vi "BUFMGR_API.vi"(0 "modpath":path, 7 "Cmd":string, 11 "error in":errorcluster) -> (4 "ImmedReplyString":string, 15 "error out":errorcluster)   [LabVIEW 2016]
uses:
  DBSHAND/private/vis/DatabaseHand_Element_Set(bool).vi
panel:
  out "caller path":path
  in  "Module vi name":string="buffermgrModule.vi"
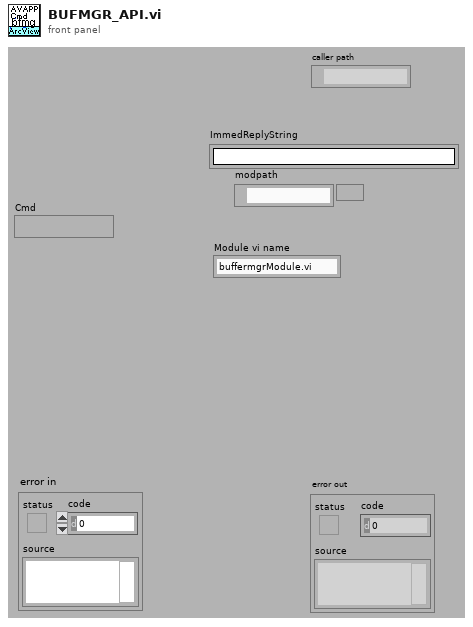
[diagram p1: front panel]
types:
  T1 = typedef "DatabaseHand_RefNum.ctl" = refnum<vi>
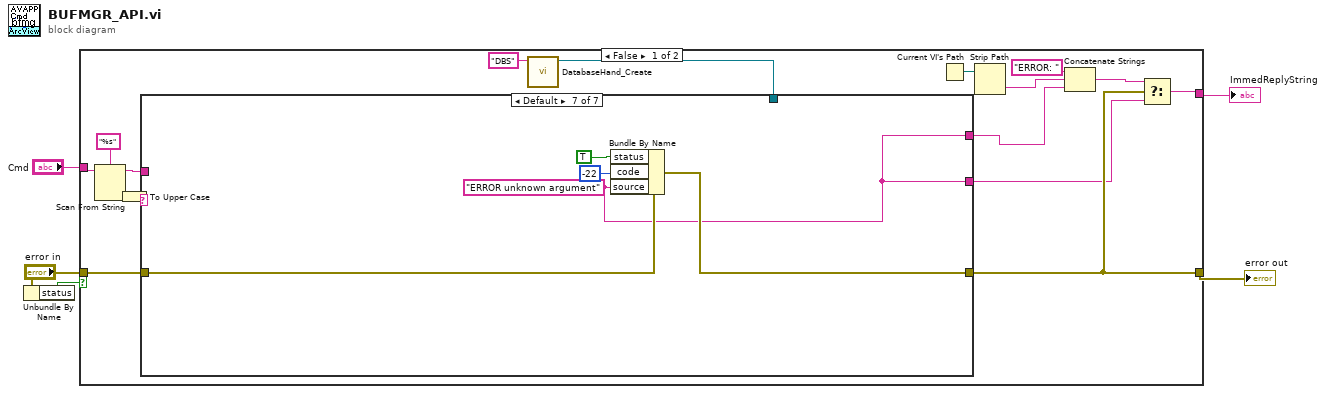
[diagram p0: block diagram]
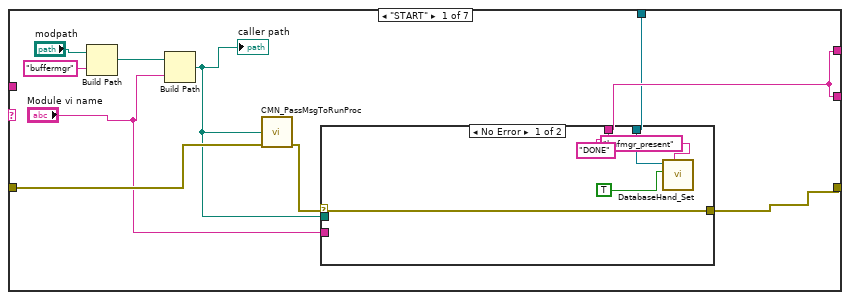
[diagram p2: hidden frame]
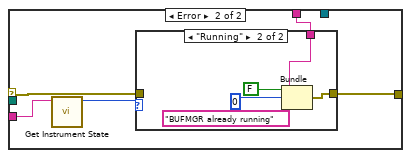
[diagram p3: hidden frame]
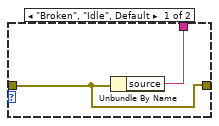
[diagram p4: hidden frame]
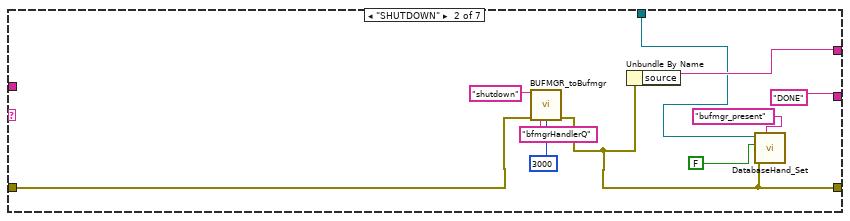
[diagram p5: hidden frame]
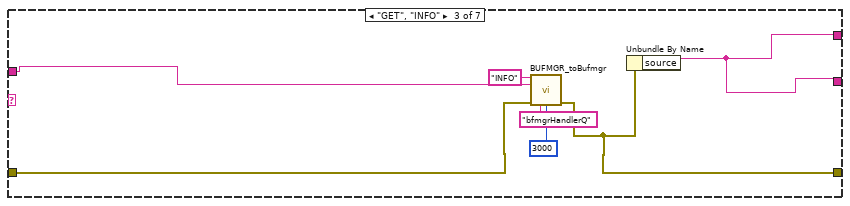
[diagram p6: hidden frame]
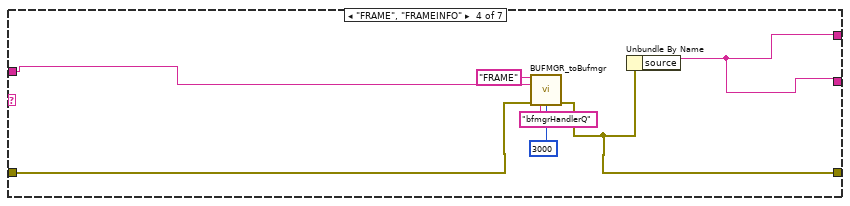
[diagram p7: hidden frame]
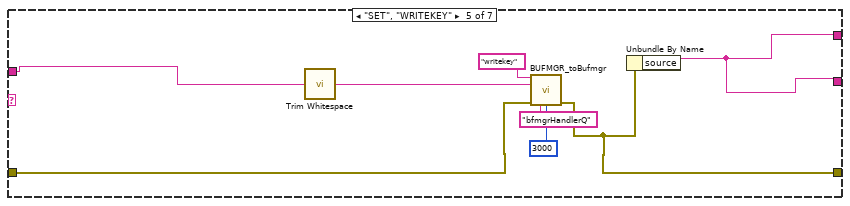
[diagram p8: hidden frame]
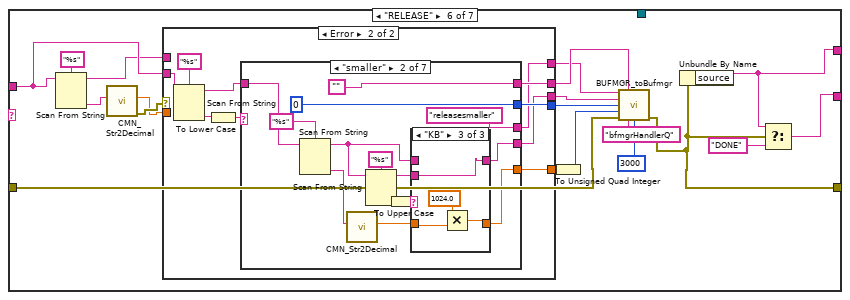
[diagram p9: hidden frame]
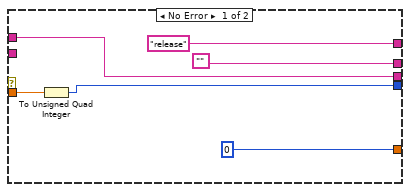
[diagram p10: hidden frame]
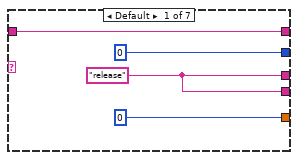
[diagram p11: hidden frame]
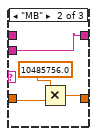
[diagram p13: hidden frame]
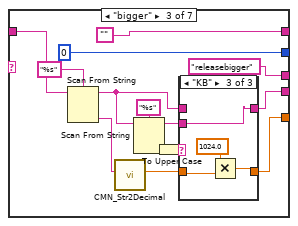
[diagram p14: hidden frame]
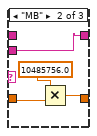
[diagram p16: hidden frame]
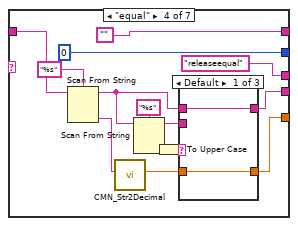
[diagram p17: hidden frame]
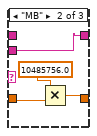
[diagram p18: hidden frame]
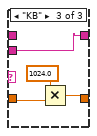
[diagram p19: hidden frame]
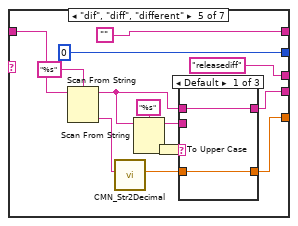
[diagram p20: hidden frame]
diagram:
  n1 = Unbundle By Name("error in") -> ("status"=w3:bool)
  n2 = case shown="False" w3 {
    tunnel: "error in" -> [w21 w229]
    tunnel: [w14 w229] -> w1
    tunnel: [w13 ""] -> w5
    tunnel: "Cmd" -> [w8 _]
    frame False {
      n3 = Scan From String(format string="%s" ("Format String"), input string=w8) -> (remaining string=w10:string, output 1=w20:string)  [unwired: 2 in, 3 out]
      n4 = To Upper Case(1:w20) -> (0:w9:string)
      n5 = call "DatabaseHand_Create.vi"("Name"="DBS") -> ("Database RefNum out"=w6:T1)  [unwired: 1 in, 9 out]
      n6 = case shown="Default" w9 {
        tunnel: w21 -> [w26 w57 w64 w71 w79 w98 w227]
        tunnel: [w30 w50 w63 w70 w78 w90 w226] -> w14
        tunnel: [w27 w55 w60 w67 w77 w89 w223] -> w12
        tunnel: [w27 "DONE" ("Message") w60 w67 w77 w88 w223] -> w11
        tunnel: w10 -> [_ _ w58 w65 w76 w82 _]
        tunnel: w6 -> [w23 w49 _ _ _ _ _]
        frame "START" {
          n7 = Build Path(base path="modpath", name or relative path="buffermgr") -> (appended path=w25:path)
          n8 = Build Path(base path=w25, name or relative path="Module vi name") -> (appended path=w22:path)
          "caller path" <- w22
          n9 = call "CMN_PassMsgToRunProc.vi"("VItoRun"=w22, "error in (no error)"=w26) -> ("error out"=w31:errorcluster)  [unwired: 1 in, 12 out]
          n10 = case shown="No Error" w31 {
            selector: w31 -> [w35 w38]
            tunnel: [w35 w39] -> w30
            tunnel: ["DONE" ("source") w40] -> w27
            tunnel: w22 -> [_ _]
            tunnel: "Module vi name" -> [_ w37]
            tunnel: w23 -> [w34 _]
            frame No Error {
              n11 = call-poly "DatabaseHand_Set.vi"("name"="bufmgr_present" ("value"), "value"=TRUE, "Database RefNum in"=w34) -> ()  [unwired: 5 in, 4 out]
            }
            frame Error {
              n12 = call <vilib>:"Get Instrument State.vi"("VI name"=w37) -> ("vi state"=w41:enum32{"Broken", "Idle", "Running"})  [unwired: 1 in, 9 out]
              n13 = case shown="\"Running\"" w41 {
                tunnel: w38 -> [w42 _]
                tunnel: [w43 w44] -> w40
                tunnel: [w42 w47] -> w39
                frame "Broken", "Idle", Default {
                  n14 = Unbundle By Name(w42) -> ("source"=w43:string)
                }
                frame "Running" {
                  w44 = "BUFMGR already running"
                  n15 = Bundle(FALSE, 0, w44) -> (w47:errorcluster)  [unwired: 1 out]
                }
              }
            }
          }
        }
        frame "SHUTDOWN" {
          n16 = call "BUFMGR_toBufmgr.vi"("command"="shutdown" ("Command"), "error in"=w57, "responseQ"="bfmgrHandlerQ", "ms timeout (-1)"=3000) -> ("error out"=w50:errorcluster)  [unwired: 4 in, 7 out]
          n17 = Unbundle By Name(w50) -> ("source"=w55:string)
          n18 = call-poly "DatabaseHand_Set.vi"("name"="bufmgr_present" ("value"), "error in (no error)"=w50, "value"=FALSE, "Database RefNum in"=w49) -> ()  [unwired: 4 in, 4 out]
        }
        frame "GET", "INFO" {
          n19 = call "BUFMGR_toBufmgr.vi"("command"="INFO", "arg"=w58, "error in"=w64, "responseQ"="bfmgrHandlerQ", "ms timeout (-1)"=3000) -> ("error out"=w63:errorcluster)  [unwired: 3 in, 7 out]
          n20 = Unbundle By Name(w63) -> ("source"=w60:string)
        }
        frame "FRAME", "FRAMEINFO" {
          n21 = call "BUFMGR_toBufmgr.vi"("command"="FRAME", "arg"=w65, "error in"=w71, "responseQ"="bfmgrHandlerQ", "ms timeout (-1)"=3000) -> ("error out"=w70:errorcluster)  [unwired: 3 in, 7 out]
          n22 = Unbundle By Name(w70) -> ("source"=w67:string)
        }
        frame "SET", "WRITEKEY" {
          n23 = call <vilib>:"Trim Whitespace.vi"("string"=w76) -> ("trimmed string"=w72:string)  [unwired: 1 in]
          n24 = call "BUFMGR_toBufmgr.vi"("command"="writekey", "arg"=w72, "error in"=w79, "responseQ"="bfmgrHandlerQ", "ms timeout (-1)"=3000) -> ("error out"=w78:errorcluster)  [unwired: 3 in, 7 out]
          n25 = Unbundle By Name(w78) -> ("source"=w77:string)
        }
        frame "RELEASE" {
          n26 = Scan From String(format string="%s", input string=w82) -> (remaining string=w81:string, output 1=w83:string)  [unwired: 2 in, 3 out]
          n27 = call "CMN_Str2Decimal.vi"("number in"=w83) -> ("error out"=w86:errorcluster, "decimal number"=w85:dbl)  [unwired: 1 in, 8 out]
          n28 = case shown="Error" w86 {
            tunnel: w85 -> [w104 _]
            tunnel: [w99 w111] -> w95
            tunnel: w82 -> [_ w114]
            tunnel: ["" w109] -> w94
            tunnel: [u64 0 w108] -> w93
            tunnel: ["release" ("command") w107] -> w92
            tunnel: [w100 w105] -> w91
            tunnel: w81 -> [w100 _]
            frame No Error {
              n29 = To Unsigned Quad Integer(1:w104) -> (0:w99:u64)
            }
            frame Error {
              n30 = Scan From String(format string="%s", input string=w114) -> (remaining string=w106:string, output 1=w110:string)  [unwired: 2 in, 3 out]
              n31 = To Lower Case(string=w110) -> (all lower case string=w112:string)
              n32 = case shown="\"smaller\"" w112 {
                tunnel: [u64 0 u64 0 u64 0 u64 0 u64 0 u64 0 u64 0] -> w111
                tunnel: w106 -> [w118 w131 w155 w179 w203 _ _]
                tunnel: [w118 "" "" "" "" w215 w219] -> w109
                tunnel: [u64 0 w120 w145 w169 w193 u64 0 u64 0] -> w108
                tunnel: [w115 "releasesmaller" ("command") "releasebigger" ("command") "releaseequal" ("command") "releasediff" ("command") "releaseall" ("command") "releaseunlocked" ("command")] -> w107
                tunnel: [w115 w121 w146 w170 w194 w215 w219] -> w105
                frame Default {
                  w115 = "release" ("command")
                }
                frame "smaller" {
                  n33 = Scan From String(format string="%s", input string=w131) -> (remaining string=w122:string, output 1=w128:string)  [unwired: 2 in, 3 out]
                  n34 = call "CMN_Str2Decimal.vi"("number in"=w128) -> ("decimal number"=w126:dbl)  [unwired: 1 in, 9 out]
                  n35 = Scan From String(format string="%s", input string=w122) -> (remaining string=w119:string, output 1=w124:string)  [unwired: 2 in, 3 out]
                  n36 = To Upper Case(1:w124) -> (0:w123:string)
                  n37 = case shown="\"KB\"" w123 {
                    tunnel: w126 -> [w133 w137 w141]
                    tunnel: w122 -> [w134 _ _]
                    tunnel: [w134 w138 w142] -> w121
                    tunnel: [w133 w135 w139] -> w120
                    tunnel: w119 -> [_ w138 w142]
                    frame Default {
                    }
                    frame "MB" {
                      n38 = Multiply(x=10485756.0, y=w137) -> (x*y=w135:dbl)
                    }
                    frame "KB" {
                      n39 = Multiply(x=1024.0, y=w141) -> (x*y=w139:dbl)
                    }
                  }
                }
                frame "bigger" {
                  n40 = Scan From String(format string="%s", input string=w155) -> (remaining string=w147:string, output 1=w152:string)  [unwired: 2 in, 3 out]
                  n41 = call "CMN_Str2Decimal.vi"("number in"=w152) -> ("decimal number"=w151:dbl)  [unwired: 1 in, 9 out]
                  n42 = Scan From String(format string="%s", input string=w147) -> (remaining string=w144:string, output 1=w149:string)  [unwired: 2 in, 3 out]
                  n43 = To Upper Case(1:w149) -> (0:w148:string)
                  n44 = case shown="\"KB\"" w148 {
                    tunnel: w151 -> [w157 w161 w165]
                    tunnel: w147 -> [w158 _ _]
                    tunnel: [w158 w162 w166] -> w146
                    tunnel: [w157 w159 w163] -> w145
                    tunnel: w144 -> [_ w162 w166]
                    frame Default {
                    }
                    frame "MB" {
                      n45 = Multiply(x=10485756.0, y=w161) -> (x*y=w159:dbl)
                    }
                    frame "KB" {
                      n46 = Multiply(x=1024.0, y=w165) -> (x*y=w163:dbl)
                    }
                  }
                }
                frame "equal" {
                  n47 = Scan From String(format string="%s", input string=w179) -> (remaining string=w171:string, output 1=w176:string)  [unwired: 2 in, 3 out]
                  n48 = call "CMN_Str2Decimal.vi"("number in"=w176) -> ("decimal number"=w175:dbl)  [unwired: 1 in, 9 out]
                  n49 = Scan From String(format string="%s", input string=w171) -> (remaining string=w168:string, output 1=w173:string)  [unwired: 2 in, 3 out]
                  n50 = To Upper Case(1:w173) -> (0:w172:string)
                  n51 = case shown="Default" w172 {
                    tunnel: w175 -> [w181 w185 w189]
                    tunnel: w171 -> [w182 _ _]
                    tunnel: [w182 w186 w190] -> w170
                    tunnel: [w181 w183 w187] -> w169
                    tunnel: w168 -> [_ w186 w190]
                    frame Default {
                    }
                    frame "MB" {
                      n52 = Multiply(x=10485756.0, y=w185) -> (x*y=w183:dbl)
                    }
                    frame "KB" {
                      n53 = Multiply(x=1024.0, y=w189) -> (x*y=w187:dbl)
                    }
                  }
                }
                frame "dif", "diff", "different" {
                  n54 = Scan From String(format string="%s", input string=w203) -> (remaining string=w195:string, output 1=w200:string)  [unwired: 2 in, 3 out]
                  n55 = call "CMN_Str2Decimal.vi"("number in"=w200) -> ("decimal number"=w199:dbl)  [unwired: 1 in, 9 out]
                  n56 = Scan From String(format string="%s", input string=w195) -> (remaining string=w192:string, output 1=w197:string)  [unwired: 2 in, 3 out]
                  n57 = To Upper Case(1:w197) -> (0:w196:string)
                  n58 = case shown="Default" w196 {
                    tunnel: w199 -> [w205 w209 w213]
                    tunnel: w195 -> [w206 _ _]
                    tunnel: [w206 w210 w214] -> w194
                    tunnel: [w205 w207 w211] -> w193
                    tunnel: w192 -> [_ w210 w214]
                    frame Default {
                    }
                    frame "MB" {
                      n59 = Multiply(x=10485756.0, y=w209) -> (x*y=w207:dbl)
                    }
                    frame "KB" {
                      n60 = Multiply(x=1024.0, y=w213) -> (x*y=w211:dbl)
                    }
                  }
                }
                frame "all" {
                  w215 = ""
                }
                frame "unlocked" {
                  w219 = ""
                }
              }
            }
          }
          n61 = To Unsigned Quad Integer(1:w93) -> (0:w80:u64)
          n62 = call "BUFMGR_toBufmgr.vi"("command"=w92, "bufname"=w94, "arg"=w91, "bufpointer"=w95, "bufsize"=w80, "error in"=w98, "responseQ"="bfmgrHandlerQ", "ms timeout (-1)"=3000) -> ("error out"=w90:errorcluster)  [unwired: 7 out]
          n63 = Unbundle By Name(w90) -> ("source"=w89:string)
          n64 = Select(t=w89, s=w90, f="DONE") -> (s? t:f=w88:string)
        }
        frame Default {
          w223 = "ERROR unknown argument" ("source")
          n65 = Bundle By Name(cluster=w227, "status"=TRUE, "code"=-22, "source"=w223) -> (w226:errorcluster)
        }
      }
      n66 = Current VI's Path() -> (path=w17:path)
      n67 = Strip Path(path=w17) -> (name=w16:string)  [unwired: 1 out]
      n68 = Concatenate Strings("ERROR: ", w16, w12) -> (w15:string)
      n69 = Select(t=w15, s=w14, f=w11) -> (s? t:f=w13:string)
    }
    frame True {
    }
  }
  "error out" <- w1
  "ImmedReplyString" <- w5
